vi "Create Shared Resources.vi"(8 "error in":errorcluster, 10 "custom device ref":T1=18446744073709551615 format="%.0x", 11 "Shared Resources Factory in":refnum<class "Shared Resources Factory.lvclass">) -> (0 "error out":errorcluster, 2 "shared resources":refnum<class "Shared Resources.lvclass">, 3 "Shared Resources Factory out":refnum<class "Shared Resources Factory.lvclass">)   [LabVIEW 2020, in "AIM ARINC 664 Engine.lvlib" / "Implementation.lvlib" / "Shared Resources Factory.lvclass"]
uses:
  Shared Resources Factory.lvclass
  <vilib>/NI VeriStand/Custom Device API/Custom Device Item Ref.ctl
  Interfaces/Shared Resources/Shared Resources.lvclass
  Shared Resources/Shared Resources.lvclass
  C:/Users/Administrator/Desktop/GIT/niveristand-aim-arinc664-custom-device/Source/Custom Device Support/Engine/Interfaces/Shared Resources/Shared Resources.lvclass
  Scripting/AIM ARINC 664 Scripting.lvlib
  <vilib>/NI VeriStand/Custom Device API/Custom Device API.lvlib
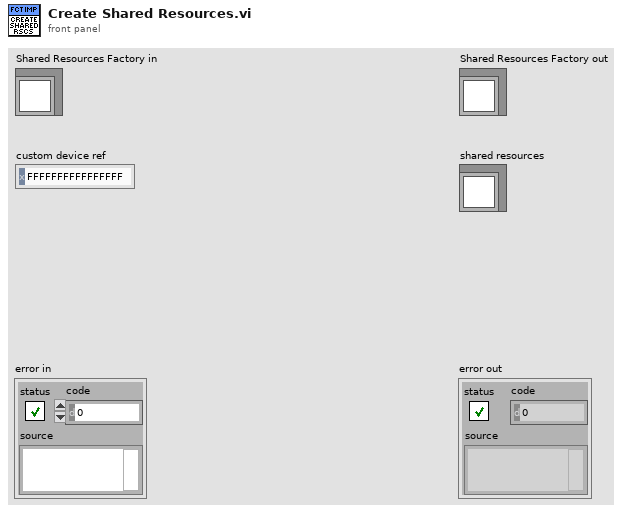
[diagram p1: front panel]
types:
  T1 = typedef "Custom Device API.lvlib/Custom Device Item Ref.ctl" = u64
  T2 = typedef "AIM ARINC 664 Import.lvlib/board_setup.ctl" = cluster{"boardId":u32, "portSpeed":u32, "portConfig":u32}
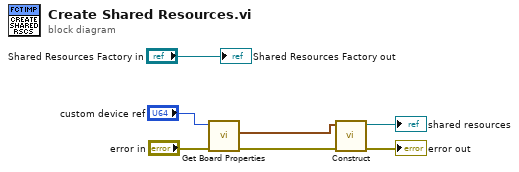
[diagram p0: block diagram]
diagram:
  n1 = call "Get Board Properties.vi"("error in"="error in", "custom device ref"="custom device ref") -> ("error out"=w2:errorcluster, "board properties out"=w1:T2)  [unwired: 7 in, 1 out]
  n2 = call "Construct.vi"("error in"=w2, "board properties in"=w1) -> ("error out"=→"error out":errorcluster, "Shared Resources out"=→"shared resources":refnum<class "Shared Resources.lvclass">)  [unwired: 8 in]
  "Shared Resources Factory out" <- "Shared Resources Factory in"
